vi "Kafka_Consume.vi"(7 "Offset Index":i64, 8 "error in (no error)":errorcluster, 9 "Max Events":i64=-1, 10 "Kafka Offset":enum16{"Beginning", "End", "Offset"}(ring), 11 "Consumer Handle":string="localhost:9092") -> (0 "error out":errorcluster, 1 "Kafka Events":T1[](array[typedef]), 2 "Num Events":i64=-1, 3 "Consumer Handle":string)   [LabVIEW 2019]
uses:
  KafkaConsumerEvent.ctl
  VS2017/KafkaLVLib/x64/Debug/KafkaLVLib.dll
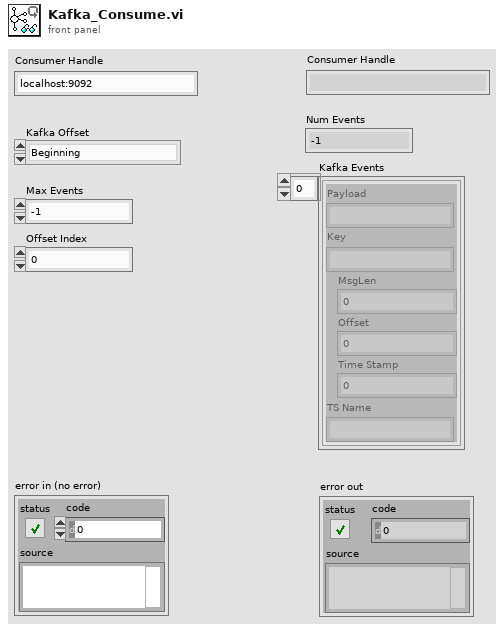
[diagram p1: front panel]
types:
  T1 = typedef "KafkaConsumerEvent.ctl" = cluster{"Payload":string, "Key":string, "MsgLen":u64, "Offset":i64, "Time Stamp":i64, "TS Name":string}
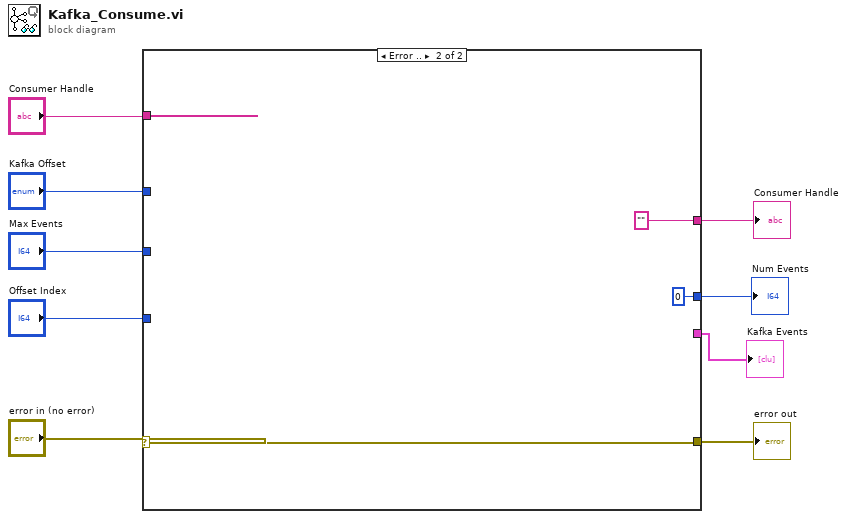
[diagram p0: block diagram]
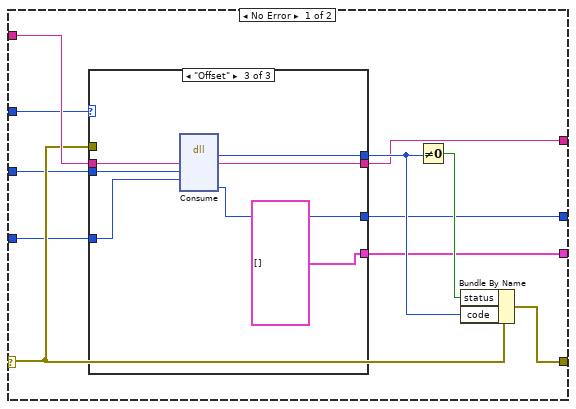
[diagram p2: hidden frame]
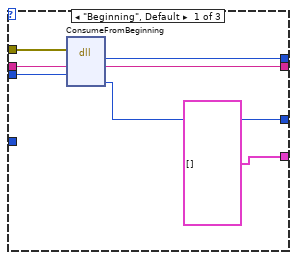
[diagram p3: hidden frame]
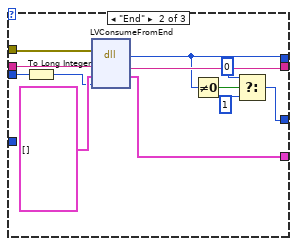
[diagram p4: hidden frame]
diagram:
  n1 = case shown="Error .." "error in (no error)" {
    selector: "error in (no error)" -> [w16 w48]
    tunnel: "Consumer Handle" -> [w17 _]
    tunnel: [w18 w48] -> w7
    tunnel: [w15 "" ("consumerHandle")] -> w6
    tunnel: "Max Events" -> [w14 _]
    tunnel: "Kafka Offset" -> [w13 _]
    tunnel: "Offset Index" -> [w12 _]
    tunnel: [w11 i64 0 ("numEvents")] -> w2
    tunnel: [w10 _] -> w1
    frame No Error {
      n2 = case shown="\"Offset\"" w13 {
        tunnel: [w27 w35 w41] -> w19
        tunnel: w17 -> [w26 w39 w43]
        tunnel: w16 -> [w25 w37 _]
        tunnel: [w24 w38 w42] -> w15
        tunnel: w14 -> [w23 w30 w45]
        tunnel: w12 -> [_ _ w46]
        tunnel: [w22 w31 w44] -> w11
        tunnel: [T1[] [] w28 T1[] []] -> w10
        frame "Beginning", Default {
          n3 = dll-call lib="C:/Users/schandho/OneDrive - National Instruments/Research/Virtualization/SemiADV/KafkaLVLib/VS2017/KafkaLVLib/x64/Debug/KafkaLVLib.dll" fn="ConsumeFromBeginning"(error in=w25, "consumerhandle"=w26, "maxEvents"=w23) -> ("error"=w27:i32, "consumerhandle"=w24:string, "numEvents"=w22:i64)  [unwired: 4 in, 2 out]
        }
        frame "End" {
          n4 = To Long Integer(number=w30) -> (32bit integer=w29:i32)
          n5 = dll-call lib="C:/Users/schandho/OneDrive - National Instruments/Research/Virtualization/SemiADV/KafkaLVLib/VS2017/KafkaLVLib/x64/Debug/KafkaLVLib.dll" fn="LVConsumeFromEnd"(error in=w37, "consumerhandle"=w39, "event"=T1[] [] ("Events 2"), "count"=w29) -> ("error"=w35:i32, "consumerhandle"=w38:string, "event"=w28:T1[])  [unwired: 3 in, 2 out]
          n6 = Not Equal To 0?(x=w35) -> (x != 0?=w34:bool)
          n7 = Select(t=i64 0 ("numEvents"), s=w34, f=i64 1 ("numEvents")) -> (s? t:f=w31:i64)
        }
        frame "Offset" {
          n8 = dll-call lib="C:/Users/schandho/OneDrive - National Instruments/Research/Virtualization/SemiADV/KafkaLVLib/VS2017/KafkaLVLib/x64/Debug/KafkaLVLib.dll" fn="Consume"("consumerhandle"=w43, "maxEvents"=w45, "offset"=w46) -> ("error"=w41:i32, "consumerhandle"=w42:string, "numEvents"=w44:i64)  [unwired: 6 in, 2 out]
        }
      }
      n9 = Not Equal To 0?(x=w19) -> (x != 0?=w20:bool)
      n10 = Bundle By Name(cluster=w16, "status"=w20, "code"=w19) -> (w18:errorcluster)
    }
    frame Error {
    }
  }
  "error out" <- w7
  "Consumer Handle" <- w6
  "Num Events" <- w2
  "Kafka Events" <- w1
